vi "Dashboard Main.vi"() -> ()   [LabVIEW 2014]
uses:
  <vilib>/event_ctls.llb/eventvkey.ctl
  <vilib>/Rock Robotics/WPI/Dashboard/WPI_DashboardLogging Global.vi
  <vilib>/Utility/config.llb/Write Key (String).vi
  <vilib>/Utility/config.llb/Write Key (I32).vi
  <vilib>/Utility/config.llb/NI_LVConfig.lvlib
panel:
  out "Camera Image":T1(plugin-control)
  in  "TCP":refnum<k5>
  in  "Rec Mode":enum32{"Stop", "Record", "Playback"}(radio)
  in  "Vision":u16(ring) items=["Camera Off", "USB Camera SW", "USB Camera HW", "IP Camera"]
  out "Camera IP":string
  out "Image Message":string="Timeout in Camera Communications"
  in  "Dashboard Tab":T2(tab)
  in  "Drivetrain D":dbl
  in  "Drivetrain I":dbl
  in  "Drivetrain P":dbl
  in  "Camera Settings":T3={"Frame Rate"=30, "Compression"=30, "Size"=1} {"Frame Rate" scale=1.0..30.0; "Size" items=["640x480", "320x240", "160x120"]}
  out "MotorChart R":cluster{"Numeric":dbl, "Numeric":dbl}(graph)
  out "MotorChart L":T4(graph)
  out "MotorSliders R":cluster{"MotorSlide1":dbl, "MotorSlide2":dbl} {"MotorSlide2" scale=-1.0..1.0 scale format="%#_2e"; "MotorSlide1" scale=-1.0..1.0 scale format="%#_2e"}
  out "MotorSliders L":T5 {"MotorSlide4 2" scale=0.0..14.0 scale format="%#_2e"; "MotorSlide2" scale=-1.0..1.0 scale format="%#_2e"; "MotorSlide1" scale=-1.0..1.0 scale format="%#_2e"}
  out "Gyro":dbl(knob) scale=0.0..360.0
  out "JS1 Z":dbl(slide) scale=-1.0..1.0 scale format="%#_2e"
  out "JS1 Graph":cluster{"X":dbl, "Y":dbl}[](graph)
  out "JS1 Buttons":T6
  out "JS2 Z":dbl(slide) scale=-1.0..1.0 scale format="%#_2e"
  out "JS2 Graph":cluster{"X":dbl, "Y":dbl}[](graph)
  out "JS2 Buttons":T6
  out "Mode":T7(ring)=enum."Auto Disabled"
  in  "DB Camera Config":bool
  out "fps":dbl format="%#.1g"
  out "Mbps":dbl format="%#.1g"
  out "Mbps 2":bool
  in  "Test Slider":dbl(slide) scale=0.0..100.0 scale format="%#_3g"
  in  "On/Off":bool caption="Solenoid"
  in  "Test Name":u16(ring) items=["Select the test to run...", "Example Test", "-------------------------------", "List of tests is built in robot code.", "Replace with your own automated tests."]
  in  "Test Tree":string(tree)
  in  "Motor":cluster{"Value":dbl, "Enable":bool} {"Value" scale=-1.0..1.0 scale format="%#_3g"}
  out "Progress":T8 {"Test Progress" scale=0.0..100.0}
  in  "Rev/Fwd":cluster{"Forward":bool, "Reverse":bool}
  in  "Test Ring":u16(ring) items=["Monochrome", "Color"]
  in  "Listbox":i32(listbox)
  out "Tree":string(tree)
  # "Left"
  # "Front"
  # "Right"
  # "Battery"
  # "This tab is a great place for autonomous settings and robot-specific values.\nPlace controls and indicators inside this tab and match name to\nDashboard Variables on robot. You can also delete this comment."
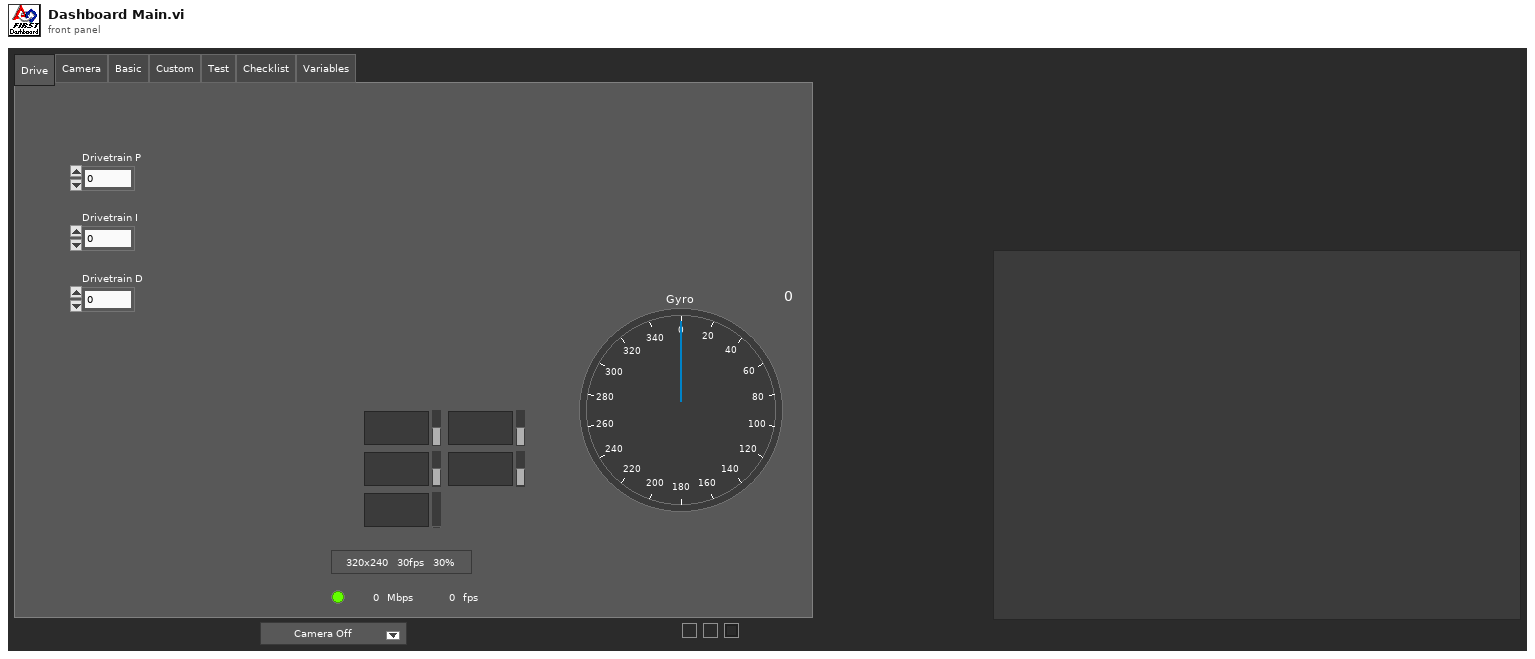
[diagram p1: front panel]
types:
  T1 = typedef "IMAQ Image.ctl" = refnum<image>
  T2 = enum32{"Drive", "Camera", "Basic", "Custom", "Test", "Checklist", "Variables"}
  T3 = cluster{"Frame Rate":i32, "Compression":i32, "Size":u16}
  T4 = cluster{"Numeric":dbl, "Numeric":dbl, "Battery V":dbl}
  T5 = cluster{"MotorSlide1":dbl, "MotorSlide2":dbl, "MotorSlide4 2":dbl}
  T6 = cluster{bool, bool, bool, bool, bool, bool, bool, bool, bool, bool, bool, bool}
  T7 = enum8{"Tele-Op Disabled", "Tele-Op Enabled", "Auto Disabled", "Auto Enabled", "Test Disabled", "Test Enabled", "Disconnected", "No Code", "E-Stop"}
  T8 = cluster{"Test Progress":u8, "Test Progress Text":string}
  T9 = typedef "Image Type" = u32
  T10 = cluster{"Error Strings":string, "Disable Counts":cluster{u16, u16}, "Rail Faults":cluster{u16, u16, u16}, "Robot IP":string, "DB Mode":u8, "Event Info":cluster{"Name":string, "Type":u8, "Number":u16, "Replay":u8}, "Camera Addr":string}
  T11 = cluster{"Storage":cluster{"Disk Free":u64, "RAM Block":u32, "RAM free":u32}, "CPU Utilization":cluster{"CPU % ISR":sgl, "CPU % Time Crit":sgl, "CPU % Timed Str":sgl, "CPU % High":sgl, "CPU % Above":sgl, "CPU % Normal":sgl, "CPU % Low":sgl}, "CAN":cluster{"% Bus Utilization":sgl, "Bus Off Cnt":u32, "TX_FIFO Full Cnt":u32, "Receive Error Cnt":u8, "Transmit Error Cnt":u8}, "HID":cluster{"HID Outputs":u32, "Rumble Low":u16, "Rumble High":u16}[]}
  T12 = cluster{"Status bits":cluster{"Test Mode":bool, "Autonomous":bool, "Enabled":bool, "Code Start":bool, "Brownout":bool, "Reserved 2":bool, "Reserved 3":bool, "E-Stop":bool}, "Code Trace":cluster{"Disabled":bool, "TeleOp":bool, "Auto":bool, "Test":bool}, "Controller Type":enum16{"unknown", "cRIO", "roboRio"}, "Code?":enum16{"unknown", "noCode", "code"}, "Battery V":dbl}
  T13 = cluster{"Control Bits":cluster{"TestMode":bool, "Autonomous":bool, "Enabled":bool, "FMS Present":bool, bool, bool, bool, "E-Stop":bool}, "Team Station ":u8, "Countdown":sgl, "Joystick Values":cluster{"Axes":dbl[], "Buttons":bool[], "POVs":i16[]}[]}
  T14 = cluster{"Axes":dbl[], "Buttons":bool[], "POVs":i16[]}[]
  T15 = cluster{"Axes":dbl[], "Buttons":bool[], "POVs":i16[]}
  T16 = cluster{"Buttons[0]":bool, "Buttons[1]":bool, "Buttons[2]":bool, "Buttons[3]":bool, "Buttons[4]":bool, "Buttons[5]":bool, "Buttons[6]":bool, "Buttons[7]":bool, "Buttons[8]":bool, "Buttons[9]":bool, "Buttons[10]":bool, "Buttons[11]":bool}
  T17 = typedef "NI_LVConfig.lvlib/Config Data RefNum.ctl" = refnum<k1>
  T18 = cluster{"Operation":enum16{"Update", "Clear"}, "Color Box":u32}[]
  T19 = typedef "eventvkey.ctl" = enum16{"ASCII", "Enter", "Return", "Shift", "Ctrl", "Alt", "Cmd", "Opt", "Caps", "NumLock", "Clear", "Break", "Up", "Down", "Left", "Right", "Insert", "Delete", "Home", "End", "PageUp", "PageDown", "Escape", "Help", "Pause", "ScrollLock", "F1", "F2", "F3", "F4", "F5", "F6", "F7", "F8", "F9", "F10", "F11", "F12", "F13", "F14", "F15", "F16", "F17", "F18", "F19", "F20", "F21", "F22", "F23", "F24", "Play", "VolumeUp", "VolumeDown", "Mute", "Two Byte Char"}
  T20 = cluster{"Image Size":bool, "Image Type":bool, "Pixel Value":bool, "ROI Information":bool, "Zoom Factor":bool}
  T21 = enum8{"Enabled", "Disabled", "Disabled and Grayed Out"}
  T22 = cluster{"Operation":enum16{"Update", "Clear"}, "Color Box":u32}
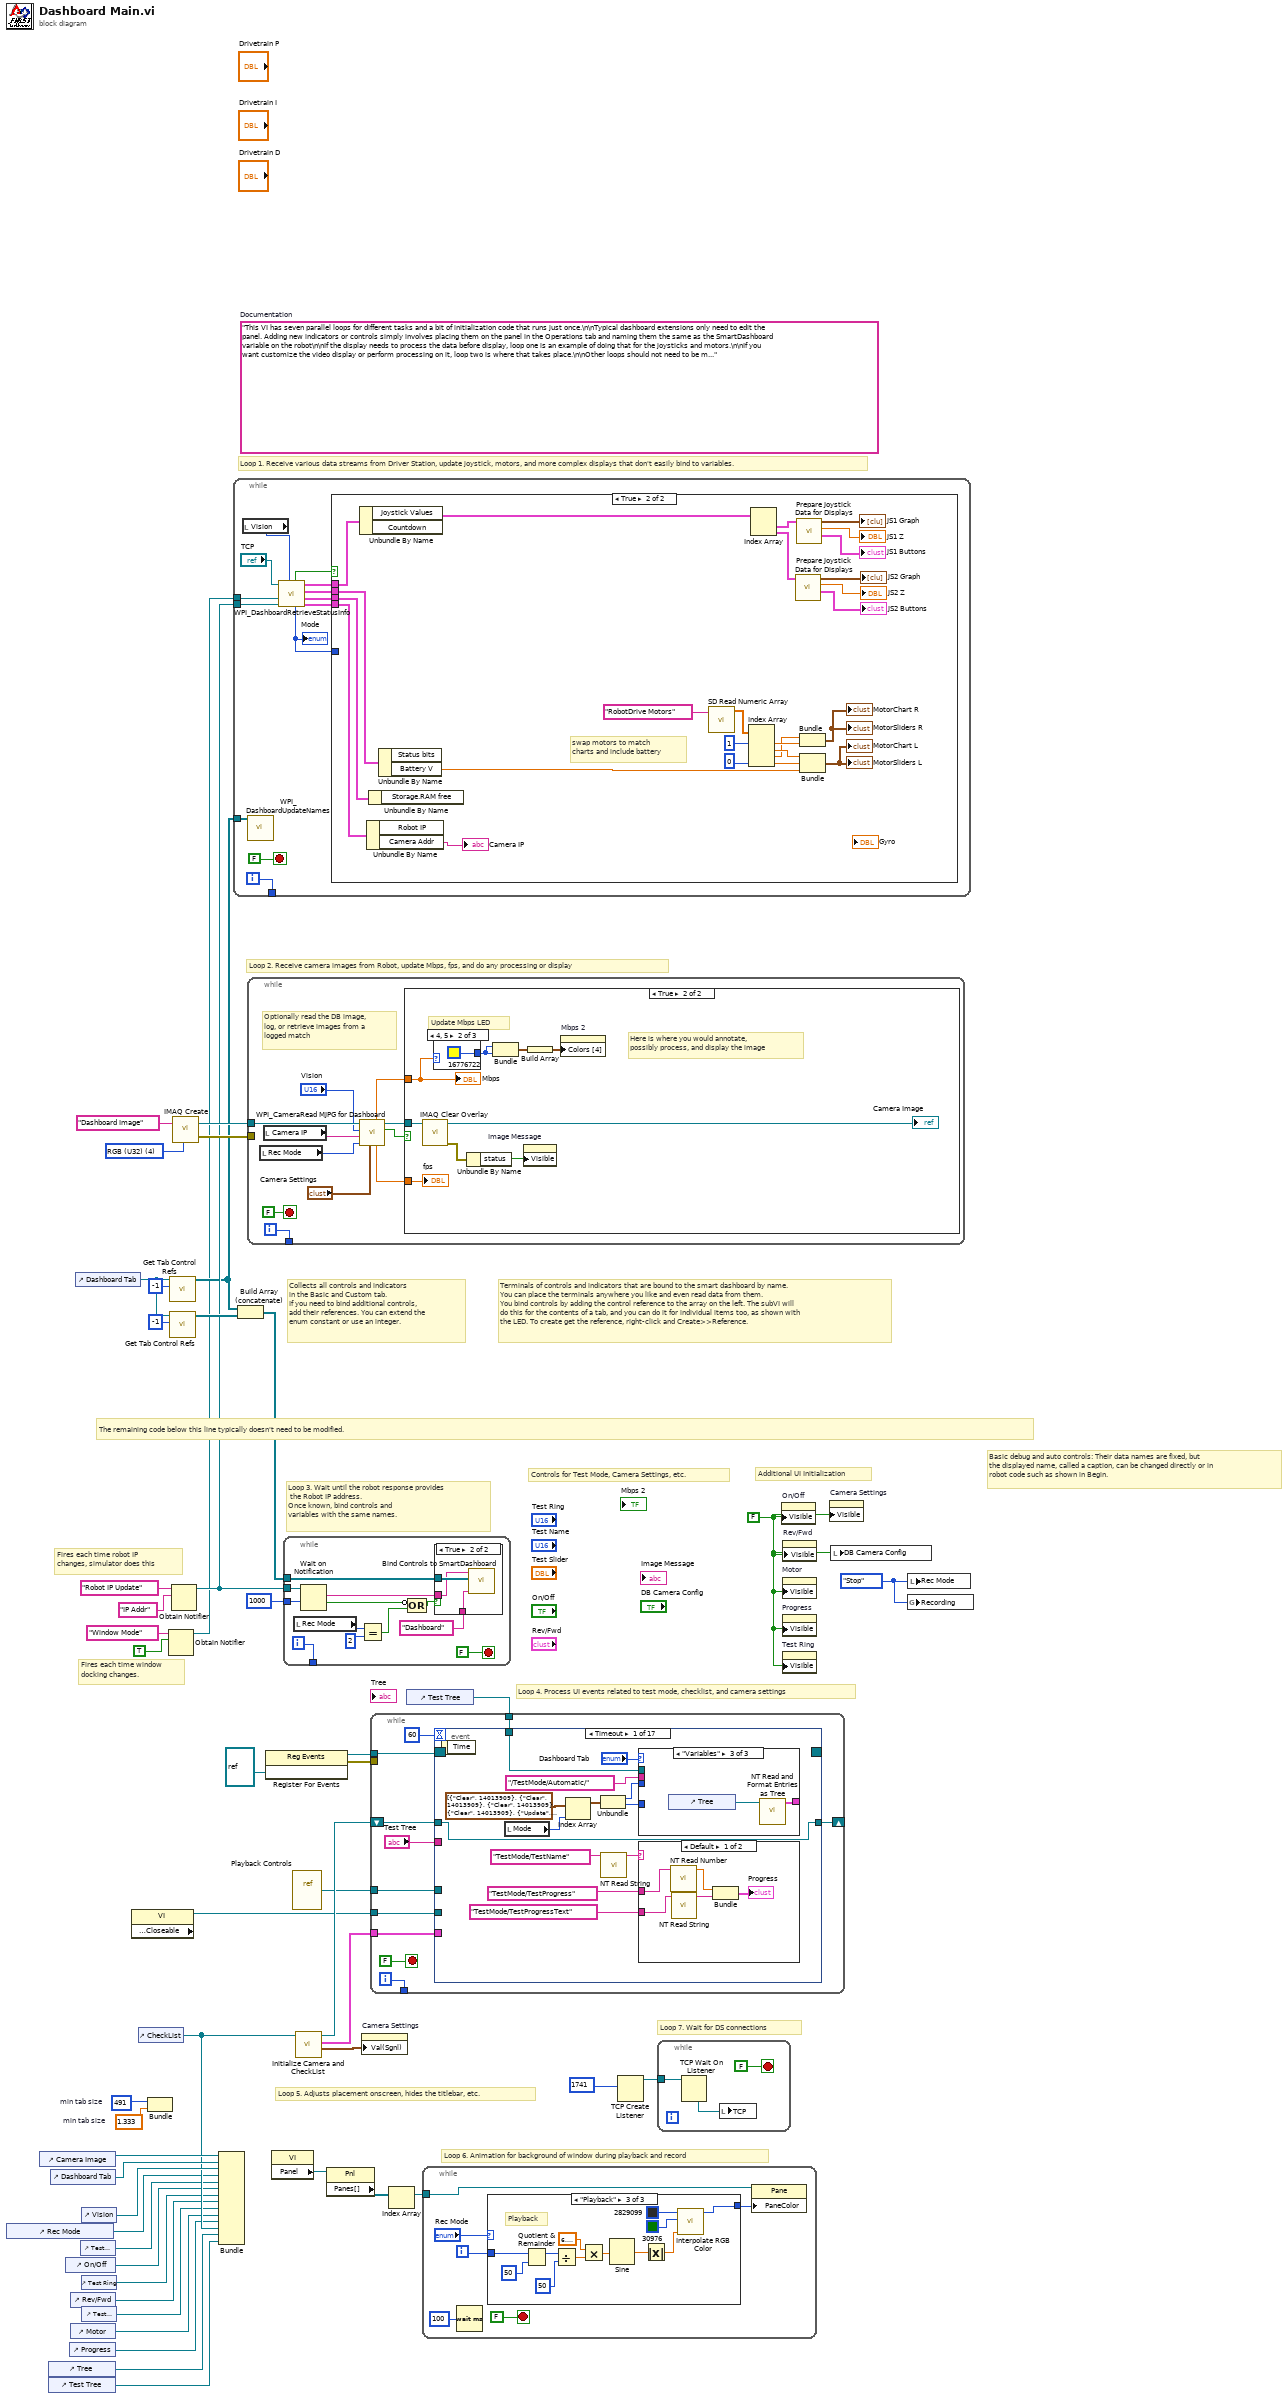
[diagram p0: block diagram]
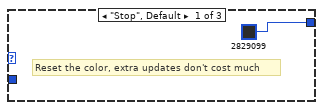
[diagram p3: hidden frame]
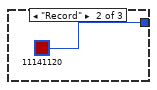
[diagram p4: hidden frame]
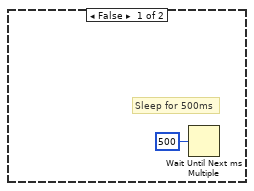
[diagram p6: hidden frame]
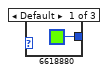
[diagram p7: hidden frame]
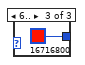
[diagram p8: hidden frame]
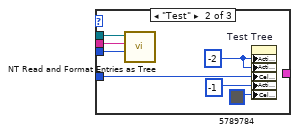
[diagram p10: hidden frame]
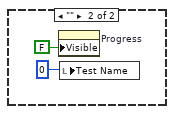
[diagram p11: hidden frame]
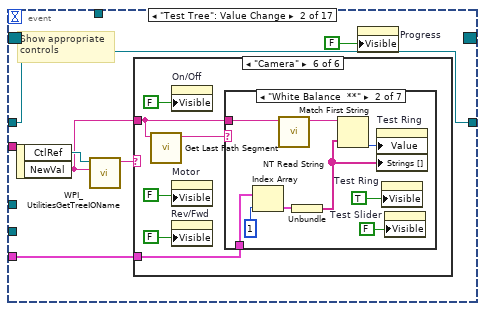
[diagram p12: hidden frame]
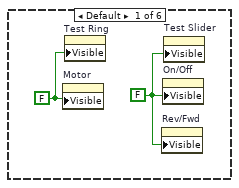
[diagram p13: hidden frame]
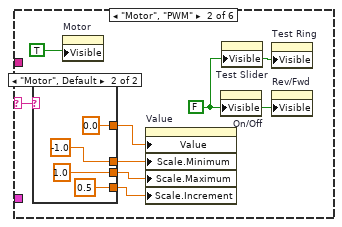
[diagram p14: hidden frame]
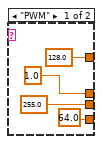
[diagram p15: hidden frame]
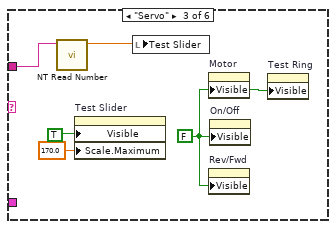
[diagram p16: hidden frame]
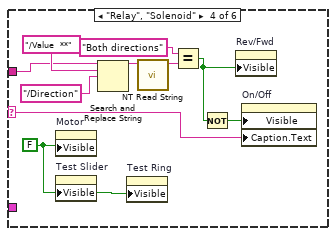
[diagram p17: hidden frame]
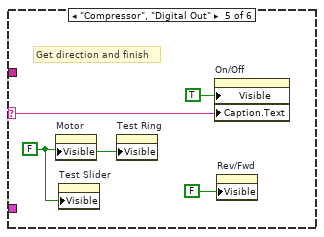
[diagram p18: hidden frame]
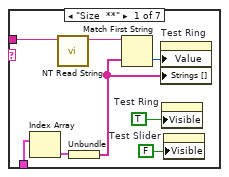
[diagram p19: hidden frame]
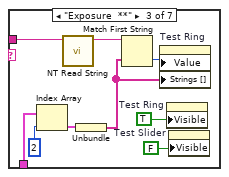
[diagram p20: hidden frame]
diagram:
  w21 = 491  # min tab size
  w20 = 1.333  # min tab size
  w29 = enum32{"Stop", "Record", "Playback"}."Stop" ("Rec Mode")
  w8 = FALSE ("Visible")
  (unwired) "This VI has seven parallel loops for different tasks and a bit of initialization code that runs just once.\n\nTypical dashboard extensions only need to edit the panel. Adding new indicators or controls simply involves placing them on the panel in the Operations tab and naming them the same as the SmartDashboard variable on the robot\n\nIf the display needs to process the data before display, loop one is an example of doing that for the joysticks and motors.\n\nIf you want customize the video display or perform processing on it, loop two is where that takes place.\n\nOther loops should not need to be modified. They are pretty standard, and document the task they perform."  # Documentation
  w49 = T9 4 items=["Grayscale (U8)", "Grayscale (I16)", "Grayscale (SGL)", "Complex (CSG)", "RGB (U32)", "HSL (U32)", "RGB (U64)"] ("Image Type")
  # "Loop 7. Wait for DS connections"
  # "Basic debug and auto controls: Their data names are fixed, but\nthe displayed name, called a caption, can be changed directly or in\nrobot code such as shown in Begin."
  # "Controls for Test Mode, Camera Settings, etc."
  # "Additional UI Initialization"
  # "Loop 6. Animation for background of window during playback and record"
  # "Fires each time robot IP\nchanges, simulator does this"
  # "Fires each time window\ndocking changes."
  # "Collects all controls and indicators\nin the Basic and Custom tab.\nIf you need to bind additional controls,\nadd their references. You can extend the\nenum constant or use an integer."
  # "The remaining code below this line typically doesn't need to be modified."
  # "Loop 4. Process UI events related to test mode, checklist, and camera settings"
  # "Terminals of controls and indicators that are bound to the smart dashboard by name.\nYou can place the terminals anywhere you like and even read data from them.\nYou bind controls by adding the control reference to the array on the left. The subVI will\ndo this for the contents of a tab, and you can do it for individual items too, as shown with\nthe LED. To create get the reference, right-click and Create>>Reference."
  # "Loop 3. Wait until the robot response provides\n the Robot IP address.\nOnce known, bind controls and\nvariables with the same names."
  # "Loop 5. Adjusts placement onscreen, hides the titlebar, etc."
  # "Loop 1. Receive various data streams from Driver Station, update joystick, motors, and more complex displays that don't easily bind to variables."
  # "Loop 2. Receive camera images from Robot, update Mbps, fps, and do any processing or display"
  n1 = control-ref of="Rec Mode"() -> (w14:refnum<vi>)
  n2 = control-ref of="Camera Image"() -> (w24:refnum<vi>)
  n3 = control-ref of="Tree"() -> (w18:refnum<vi>)
  n4 = control-ref of="Test Tree"() -> (w17:refnum<vi>)
  n5 = control-ref of="Dashboard Tab"() -> (w23:refnum<vi>)
  n6 = control-ref of="On/Off"() -> (w12:refnum<vi>)
  n7 = control-ref of="Progress"() -> (w9:refnum<vi>)
  n8 = control-ref of="Rev/Fwd"() -> (w10:refnum<vi>)
  n9 = control-ref of="Motor"() -> (w15:refnum<vi>)
  n10 = control-ref of="Dashboard Tab"() -> (w27:refnum<vi>)
  n11 = control-ref of="Test Slider"() -> (w13:refnum<vi>)
  n12 = control-ref of="Vision"() -> (w22:refnum<vi>)
  n13 = control-ref of="Test Ring"() -> (w11:refnum<vi>)
  n14 = control-ref of="Test Name"() -> (w16:refnum<vi>)
  n15 = property class="VI" props=["Front Panel.Closeable"]() -> (reference out=w28:refnum<vi>)  [unwired: 2 in, 2 out]
  n16 = control-ref of="CheckList"() -> (w19:refnum<vi>)
  n17 = Bundle("min tab size"=w21, "min tab size"=w20) -> ()  [unwired: 1 in, 1 out]
  n18 = Obtain Notifier(name (unnamed)="Window Mode", notification data type=TRUE) -> (notifier out=w5:refnum<notifier>)  [unwired: 2 in, 2 out]
  n19 = call <vilib>:"Get Tab Control Refs.vi"("Page Index"=-1, "TabControl in"=w27) -> ("ControlsOnPage"=w6:refnum<vi>[])  [unwired: 9 in]
  n20 = call <vilib>:"Get Tab Control Refs.vi"("Page Index"=-1, "TabControl in"=w27) -> ("ControlsOnPage"=w26:refnum<vi>[])  [unwired: 9 in]
  n21 = Obtain Notifier(name (unnamed)="Robot IP Update", notification data type="IP Addr" ("name (unnamed)")) -> (notifier out=w7:refnum<notifier>)  [unwired: 2 in, 2 out]
  n22 = call "IMAQ Create"("Image Name"="Dashboard Image", "Image Type"=w49) -> ("New Image"=w47:T1, "error out"=w46:errorcluster)  [unwired: 2 in, 1 out]
  n23 = Bundle("Camera Image"=w24, "Dashboard Tab"=w23, "Vision"=w22, "Rec Mode"=w14, "Test Slider"=w13, "On/Off"=w12, "Test Ring"=w11, "Rev/Fwd"=w10, "Test Name"=w16, "Motor"=w15, "Progress"=w9, "CheckList"=w19, "Tree"=w18, "Test Tree"=w17) -> ()  [unwired: 1 in, 1 out]
  n24 = while {
    tunnel: [w61] -> _
    tunnel: w7 -> [w55]
    tunnel: w6 -> [w54]
    tunnel: w5 -> [w50]
    i -> [w61]
    stop <- FALSE stop-if-true
    n25 = local read "Vision"() -> (w52:u16)
    n26 = call <vilib>:"WPI_DashboardUpdateNames.vi"("Controls on Tab"=w54) -> ()  [unwired: 11 in]
    n27 = call <vilib>:"WPI_DashboardRetrieveStatusInfo.vi"("Vision"=w52, "Binding Refnum"=w55, "Window Mode Notifier"=w50, "TCP Cnx"="TCP") -> ("Power and Errors"=w56:T10, "Robot Metrics"=w59:T11, "Status Info"=w60:T12, "Control Info"=w57:T13, "Robot Mode"=w53:T7, "Process?"=w58:bool)  [unwired: 2 in]
    "Mode" <- w53
    n28 = case shown="True" w58 {
      tunnel: w60 -> [_ w87]
      tunnel: w59 -> [_ w86]
      tunnel: w57 -> [_ w85]
      tunnel: w56 -> [_ w84]
      tunnel: w53 -> [_ _]
      frame False {
      }
      frame True {
        # "swap motors to match\ncharts and include battery"
        n29 = Unbundle By Name(w85) -> ("Joystick Values"=w72:T14)  [unwired: 1 out]
        n30 = Unbundle By Name(w84) -> ("Camera Addr"=→"Camera IP":string)  [unwired: 1 out]
        n31 = Unbundle By Name(w86) -> ()  [unwired: 1 out]
        n32 = Unbundle By Name(w87) -> ("Battery V"=w73:dbl)  [unwired: 1 out]
        n33 = call <vilib>:"SD Read Numeric Array.vi"("Name"="RobotDrive Motors") -> ("Numeric Array"=w75:dbl[])  [unwired: 8 in, 2 out]
        n34 = Index Array(array=w75, index #1=1, index #4=0) -> (element #1=w79:dbl, element #2=w80:dbl, element #3=w78:dbl, element #4=w83:dbl)  [unwired: 2 in]
        n35 = Index Array(array=w72) -> (element #1=w71:T15, element #2=w66:T15)  [unwired: 2 in]
        n36 = call "Prepare Joystick Data for Displays.vi"("Joystick Values"=w66) -> ("Buttons"=→"JS2 Buttons":T16, "Z Axis"=→"JS2 Z":dbl, "Cartesian Data"=→"JS2 Graph":cluster{"X axis":dbl, "X axis":dbl}[])  [unwired: 8 in]
        n37 = call "Prepare Joystick Data for Displays.vi"("Joystick Values"=w71) -> ("Buttons"=→"JS1 Buttons":T16, "Z Axis"=→"JS1 Z":dbl, "Cartesian Data"=→"JS1 Graph":cluster{"X axis":dbl, "X axis":dbl}[])  [unwired: 8 in]
        n38 = Bundle("Numeric"=w78, "Numeric"=w79) -> (→"MotorChart R" →"MotorSliders R":cluster{"Numeric":dbl, "Numeric":dbl})  [unwired: 1 in]
        n39 = Bundle("Numeric"=w80, "Numeric"=w83, "Battery V"=w73) -> (→"MotorChart L" →"MotorSliders L":T4)  [unwired: 1 in]
      }
    }
  }
  n40 = Build Array (concatenate)(w6, w26) -> (w25:refnum<vi>[])
  n41 = while {
    tunnel: w47 -> [w96]
    tunnel: w46 -> [_]
    tunnel: [w97] -> _
    i -> [w97]
    stop <- FALSE stop-if-true
    # "Optionally read the DB image,\nlog, or retrieve images from a\nlogged match"
    n42 = local read "Rec Mode"() -> (w90:enum32{"Stop", "Record", "Playback"})
    n43 = local read "Camera IP"() -> (w88:string)
    n44 = call <vilib>:"WPI_CameraRead MJPG for Dashboard.vi"("Camera Settings"="Camera Settings", "Rec Mode"=w90, "Camera IP"=w88, "Camera Mode"="Vision", "Refnum in"=w96) -> ("Active"=w94:bool, "Refnum out"=w95:T1, "FPS"=w93:dbl, "Bandwidth (Mbps)"=w92:dbl)  [unwired: 3 in]
    n45 = case shown="True" w94 {
      tunnel: w95 -> [_ w103]
      tunnel: w92 -> [_ w102]
      tunnel: w93 -> [_ w100]
      frame False {
        # "Sleep for 500ms"
        n46 = Wait Until Next ms Multiple(millisecond multiple=u32 500) -> ()  [unwired: 1 out]
      }
      frame True {
        # "Here is where you would annotate,\npossibly process, and display the image"
        # "Update Mbps LED"
        n47 = call "IMAQ Clear Overlay"("Image"=w103) -> ("error out"=w107:errorcluster, "Image Out"=→"Camera Image":T1)  [unwired: 2 in, 7 out]
        n48 = case shown="4, 5" w102 {
          tunnel: [u32 6618880 ("Color Box") u32 16776722 ("Color Box") u32 16716800 ("Color Box")] -> w104
          frame Default {
          }
          frame 4, 5 {
          }
          frame 6.. {
          }
        }
        n49 = Unbundle By Name(w107) -> ("status"=w108:bool)
        n50 = Bundle("Color Box"=w104, "Color Box"=w104) -> (w106:cluster{"Color Box":u32, "Color Box":u32})  [unwired: 1 out]
        n51 = property on="Image Message" class="Str"("Visible"=w108) -> ()  [unwired: 2 in, 2 out]
        n52 = Build Array(w106) -> (w105:cluster{"Color Box":u32, "Color Box":u32}[])
        n53 = property on="Mbps 2" class="Bool (strict)"("Colors [4]"=w105) -> ()  [unwired: 2 in, 2 out]
        "Mbps" <- w102
        "fps" <- w100
      }
    }
  }
  n54 = register-events(refnum<vi> refnum) -> (reference out=w33:refnum<event-registration>, error out=w32:errorcluster)  [unwired: 2 in]
  n55 = property class="VI"() -> ("Panel"=w36:refnum<vi>)  [unwired: 2 in, 2 out]
  n56 = while {
    tunnel: w25 -> [w123]
    tunnel: w7 -> [w121]
    tunnel: [w119] -> _
    tunnel: u32 1000 ("milliseconds to wait") -> [w118]
    i -> [w119]
    stop <- FALSE stop-if-true
    n57 = local read "Rec Mode"() -> (w114:enum32{"Stop", "Record", "Playback"})
    n58 = Wait on Notification(notifier=w121, timeout in ms (-1)=w118) -> (notification=w120:string, timed out?=w116:bool)  [unwired: 2 in, 2 out]
    n59 = Equal?(x=w114, y=u16 2 ("Rec Mode")) -> (x = y?=w115:bool)
    n60 = Compound Arithmetic op=OR(invert w116, w115) -> (w117:bool)
    n61 = case shown="True" w117 {
      tunnel: w123 -> [_ w126]
      tunnel: w120 -> [_ w125]
      tunnel: "Dashboard" -> [_ w124]
      frame False {
      }
      frame True {
        n62 = call <vilib>:"Bind Controls to SmartDashboard.vi"("Client Name"=w124, "Bound Control Refs"=w126, "Server IP Address"=w125) -> ()  [unwired: 9 in]
      }
    }
  }
  n63 = vi-ref "Playback Controls.vi"() -> (w34:refnum<vi>)
  n64 = call "Initialize Camera and CheckList.vi"("ListBox in"=w19) -> ("Cluster"=w40:cluster{"value":i32, "value":i32, "index":i32}, "Array"=w41:cluster{string[]}[], "File Refnum"=w39:T17)  [unwired: 8 in]
  n65 = property class="Pnl"(reference=w36) -> ("Panes[]"=w37:refnum<vi>[])  [unwired: 1 in, 2 out]
  n66 = property on="Camera Settings" class="Clust (strict)"("Val(Sgnl)"=w40) -> ()  [unwired: 2 in, 2 out]
  n67 = Index Array(array=w37) -> (element=w35:refnum<vi>)  [unwired: 1 in]
  n68 = control-ref of="Test Tree"() -> (w38:refnum<vi>)
  n69 = while {
    tunnel: w41 -> [w134]
    shift-right: [w133] -> _
    shift-left: w39 -> [w132]
    tunnel: [w131] -> _
    tunnel: w38 -> [w130]
    tunnel: w34 -> [w129]
    tunnel: w33 -> [w128]
    tunnel: w32 -> [_]
    tunnel: w28 -> [w127]
    i -> [w131]
    stop <- FALSE stop-if-true
    n70 = event shown="[0] Timeout" {
      selector: w128 -> [_ _ _ _ _ _ _ _ _ _ _ _ _ _ _ _ _]
      dyn-events: [_ _ _ _ _ _ _ _ _ _ _ _ _ w372 _ _ _] -> _
      timeout: u32 60 ("milliseconds to wait") -> [_ _ _ _ _ _ _ _ _ _ _ _ _ _ _ _ _]
      tunnel: w130 -> [w146 _ _ _ _ _ _ _ _ _ _ _ _ _ _ _ _]
      tunnel: "Test Tree" -> [_ _ _ _ _ _ _ _ w341 w349 w351 w355 w363 _ _ _ _]
      tunnel: w134 -> [_ w168 _ _ _ _ w305 w335 _ _ _ _ _ _ _ _ _]
      tunnel: [w142 w167 w266 w271 w279 w291 w304 w328 w340 w347 w350 w354 w362 w374 w388 w389 w399] -> w133
      tunnel: w132 -> [w142 w167 w266 w271 w279 w291 w303 w328 w340 w347 w350 w354 w362 w374 w388 w389 w399]
      tunnel: w129 -> [_ _ _ _ _ _ _ _ _ _ _ _ _ w375 _ w392 _]
      tunnel: w127 -> [_ _ _ _ _ _ _ _ _ _ _ _ _ w370 _ _ _]
      event Timeout {
        n71 = event-data() -> ()  [unwired: 1 in, 1 out]
        n72 = local read "Mode"() -> (w145:T7)
        n73 = Index Array(array=T18 [{"Operation"=enum."Clear", "Color Box"=14013909}, {"Operation"=enum."Clear", "Color Box"=14013909}, {"Operation"=enum."Clear", "Color Box"=14013909}, {"Operation"=enum."Clear", "Color Box"=14013909}, {"Operation"=enum."Update", "Color Box"=14013909}, {"Operation"=enum."Update", "Color Box"=16777215}, {"Operation"=enum."Clear", "Color Box"=14013909}, {"Operation"=enum."Clear", "Color Box"=14013909}, {"Operation"=enum."Clear", "Color Box"=14013909}], index=w145) -> (element=w140:T22)
        n74 = Unbundle(w140) -> ("Operation"=w139:enum16{"Update", "Clear"}, "Color Box"=w138:u32)
        n75 = call <vilib>:"NT Read String.vi"("Name"="TestMode/TestName") -> ("String"=w149:string)  [unwired: 9 in, 1 out]
        n76 = case shown="\"Variables\"" "Dashboard Tab" {
          tunnel: w146 -> [_ w157 _]
          tunnel: "/TestMode/Automatic/" ("Name Pattern") -> [_ w156 _]
          tunnel: w139 -> [_ w155 _]
          tunnel: [_ _ w159] -> _
          tunnel: w138 -> [_ w151 _]
          frame "Custom", Default {
          }
          frame "Test" {
            w154 = -2 ("Active Item:Row Number")
            n77 = call <vilib>:"NT Read and Format Entries as Tree.vi"("Operation"=w155, "Name Pattern"=w156, "Tree Refnum"=w157) -> ()  [unwired: 7 in, 2 out]
            n78 = property on="Test Tree" class="Tree (strict)"("Active Item Row Number"=w154, "ActiveColNum"=w154, "CellBG"=w151, "Active Item Row Number"=-1 ("Active Item:Row Number"), "CellBG"=u32 5789784 ("Color Box")) -> ()  [unwired: 2 in, 2 out]
          }
          frame "Variables" {
            n79 = control-ref of="Tree"() -> (w158:refnum<vi>)
            n80 = call <vilib>:"NT Read and Format Entries as Tree.vi"("Tree Refnum"=w158) -> ("Formatted Strings"=w159:cluster{"Name":string, "Value":string}[])  [unwired: 9 in, 1 out]
          }
        }
        n81 = case shown="Default" w149 {
          tunnel: "TestMode/TestProgress" ("Name") -> [w161 _]
          tunnel: "TestMode/TestProgressText" ("Name") -> [w160 _]
          frame Default {
            n82 = call <vilib>:"NT Read Number.vi"("Name"=w161) -> ("Numeric"=w162:dbl)  [unwired: 9 in, 1 out]
            n83 = call <vilib>:"NT Read String.vi"("Name"=w160) -> ("String"=w163:string)  [unwired: 9 in, 1 out]
            n84 = Bundle("Numeric"=w162, "String"=w163) -> (→"Progress":cluster{"Numeric":dbl, "String":string})  [unwired: 1 in]
          }
          frame "" {
            n85 = property on="Progress" class="Clust (strict)"("Visible"=FALSE) -> ()  [unwired: 2 in, 2 out]
            n86 = local write "Test Name"(u16 0) -> ()
          }
        }
      }
      event "Test Tree": Value Change {
        # "Show appropriate\ncontrols"
        n87 = event-data() -> ("CtlRef"=w171:refnum<vi>, "NewVal"=w169:string)  [unwired: 1 in]
        n88 = call <vilib>:"WPI_UtilitiesGetTreeIOName.vi"("NewVal"=w169, "TreeControl in"=w171) -> ("I/O Name"=w172:string)  [unwired: 9 in]
        n89 = case shown="\"Camera\"" w172 {
          selector: w172 -> [_ w179 _ w197 w206 _]
          tunnel: w169 -> [_ _ w194 w196 _ w213]
          tunnel: w168 -> [_ _ _ _ _ w212]
          frame Default {
            w174 = FALSE ("Visible")
            w173 = FALSE ("Visible")
            n90 = property on="Motor" class="Clust (strict)"("Visible"=w173) -> ()  [unwired: 2 in, 2 out]
            n91 = property on="Test Ring" class="Ring (strict)"("Visible"=w173) -> ()  [unwired: 2 in, 2 out]
            n92 = property on="Rev/Fwd" class="Clust (strict)"("Visible"=w174) -> ()  [unwired: 2 in, 2 out]
            n93 = property on="On/Off" class="Bool (strict)"("Visible"=w174) -> ()  [unwired: 2 in, 2 out]
            n94 = property on="Test Slider" class="Slide (strict)"("Visible"=w174) -> ()  [unwired: 2 in, 2 out]
          }
          frame "Motor", "PWM" {
            w180 = FALSE ("Visible")
            n95 = case shown="\"Motor\", Default" w179 {
              tunnel: [1.0 ("Value") -1.0 ("Value")] -> w178
              tunnel: [255.0 ("Value") 1.0 ("Value")] -> w177
              tunnel: [128.0 ("Value") 0.0 ("Value")] -> w176
              tunnel: [64.0 ("Value") 0.5 ("Value")] -> w175
              frame "PWM" {
              }
              frame "Motor", Default {
              }
            }
            n96 = property on="Motor" class="Clust (strict)"("Visible"=TRUE) -> ()  [unwired: 2 in, 2 out]
            n97 = property on="Value" class="Slide (strict)"("Value"=w176, "Scale.Minimum"=w178, "Scale.Maximum"=w177, "Scale.Increment"=w175) -> ()  [unwired: 2 in, 2 out]
            n98 = property on="On/Off" class="Bool (strict)"("Visible"=w180) -> ()  [unwired: 2 in, 2 out]
            n99 = property on="Test Slider" class="Slide (strict)"("Visible"=w180) -> ()  [unwired: 2 in, 2 out]
            n100 = property on="Test Ring" class="Ring (strict)"("Visible"=w180) -> ()  [unwired: 2 in, 2 out]
            n101 = property on="Rev/Fwd" class="Clust (strict)"("Visible"=w180) -> ()  [unwired: 2 in, 2 out]
          }
          frame "Servo" {
            w192 = FALSE ("Visible")
            n102 = call <vilib>:"NT Read Number.vi"("Name"=w194) -> ("Numeric"=w193:dbl)  [unwired: 9 in, 1 out]
            n103 = property on="Test Slider" class="Slide (strict)"("Visible"=TRUE, "Scale.Maximum"=170.0 ("Scale.Range:Maximum")) -> ()  [unwired: 2 in, 2 out]
            n104 = local write "Test Slider"(w193) -> ()
            n105 = property on="Motor" class="Clust (strict)"("Visible"=w192) -> ()  [unwired: 2 in, 2 out]
            n106 = property on="Rev/Fwd" class="Clust (strict)"("Visible"=w192) -> ()  [unwired: 2 in, 2 out]
            n107 = property on="On/Off" class="Bool (strict)"("Visible"=w192) -> ()  [unwired: 2 in, 2 out]
            n108 = property on="Test Ring" class="Ring (strict)"("Visible"=w192) -> ()  [unwired: 2 in, 2 out]
          }
          frame "Relay", "Solenoid" {
            w195 = FALSE ("Visible")
            n109 = property on="Motor" class="Clust (strict)"("Visible"=w195) -> ()  [unwired: 2 in, 2 out]
            n110 = property on="Test Slider" class="Slide (strict)"("Visible"=w195) -> ()  [unwired: 2 in, 2 out]
            n111 = Search and Replace String(input string=w196, search string="/Value  **", replace string="/Direction") -> (result string=w202:string)  [unwired: 5 in, 3 out]
            n112 = property on="Test Ring" class="Ring (strict)"("Visible"=w195) -> ()  [unwired: 2 in, 2 out]
            n113 = call <vilib>:"NT Read String.vi"("Name"=w202) -> ("String"=w200:string)  [unwired: 9 in, 1 out]
            n114 = Equal?(x="Both directions", y=w200) -> (x = y?=w198:bool)
            n115 = Not(x=w198) -> (.not. x?=w199:bool)
            n116 = property on="Rev/Fwd" class="Clust (strict)"("Visible"=w198) -> ()  [unwired: 2 in, 2 out]
            n117 = property on="On/Off" class="Bool (strict)"("Visible"=w199, "Caption.Text"=w197) -> ()  [unwired: 2 in, 2 out]
          }
          frame "Compressor", "Digital Out" {
            w205 = FALSE ("Visible")
            # "Get direction and finish"
            n118 = property on="Motor" class="Clust (strict)"("Visible"=w205) -> ()  [unwired: 2 in, 2 out]
            n119 = property on="Test Slider" class="Slide (strict)"("Visible"=w205) -> ()  [unwired: 2 in, 2 out]
            n120 = property on="Test Ring" class="Ring (strict)"("Visible"=w205) -> ()  [unwired: 2 in, 2 out]
            n121 = property on="On/Off" class="Bool (strict)"("Visible"=TRUE, "Caption.Text"=w206) -> ()  [unwired: 2 in, 2 out]
            n122 = property on="Rev/Fwd" class="Clust (strict)"("Visible"=FALSE) -> ()  [unwired: 2 in, 2 out]
          }
          frame "Camera" {
            n123 = call <vilib>:"Get Last Path Segment.vi"("String in"=w213) -> ("String out"=w214:string)  [unwired: 10 in]
            n124 = property on="On/Off" class="Bool (strict)"("Visible"=FALSE) -> ()  [unwired: 2 in, 2 out]
            n125 = property on="Motor" class="Clust (strict)"("Visible"=FALSE) -> ()  [unwired: 2 in, 2 out]
            n126 = property on="Rev/Fwd" class="Clust (strict)"("Visible"=FALSE) -> ()  [unwired: 2 in, 2 out]
            n127 = case shown="\"White Balance  **\"" w214 {
              tunnel: w213 -> [w220 w229 w238 w247 w256 _ w262]
              tunnel: w212 -> [w218 w226 w235 w244 w253 _ _]
              frame "Size  **" {
                n128 = Index Array(array=w218) -> (element=w217:cluster{string[]})  [unwired: 1 in]
                n129 = call <vilib>:"NT Read String.vi"("Name"=w220) -> ("String"=w219:string)  [unwired: 9 in, 1 out]
                n130 = Unbundle(w217) -> (w215:string[])
                n131 = Match First String(2:w215, 3:w219) -> (0:w216:i32)  [unwired: 1 out]
                n132 = property on="Test Ring" class="Ring (strict)"("Value"=w216, "Strings []"=w215) -> ()  [unwired: 2 in, 2 out]
                n133 = property on="Test Ring" class="Ring (strict)"("Visible"=TRUE) -> ()  [unwired: 2 in, 2 out]
                n134 = property on="Test Slider" class="Slide (strict)"("Visible"=FALSE) -> ()  [unwired: 2 in, 2 out]
              }
              frame "White Balance  **" {
                n135 = Index Array(array=w226, index=1) -> (element=w227:cluster{string[]})
                n136 = call <vilib>:"NT Read String.vi"("Name"=w229) -> ("String"=w228:string)  [unwired: 9 in, 1 out]
                n137 = Unbundle(w227) -> (w224:string[])
                n138 = Match First String(2:w224, 3:w228) -> (0:w223:i32)  [unwired: 1 out]
                n139 = property on="Test Ring" class="Ring (strict)"("Value"=w223, "Strings []"=w224) -> ()  [unwired: 2 in, 2 out]
                n140 = property on="Test Ring" class="Ring (strict)"("Visible"=TRUE) -> ()  [unwired: 2 in, 2 out]
                n141 = property on="Test Slider" class="Slide (strict)"("Visible"=FALSE) -> ()  [unwired: 2 in, 2 out]
              }
              frame "Exposure  **" {
                n142 = Index Array(array=w235, index=2) -> (element=w236:cluster{string[]})
                n143 = call <vilib>:"NT Read String.vi"("Name"=w238) -> ("String"=w237:string)  [unwired: 9 in, 1 out]
                n144 = Unbundle(w236) -> (w232:string[])
                n145 = Match First String(2:w232, 3:w237) -> (0:w233:i32)  [unwired: 1 out]
                n146 = property on="Test Ring" class="Ring (strict)"("Value"=w233, "Strings []"=w232) -> ()  [unwired: 2 in, 2 out]
                n147 = property on="Test Ring" class="Ring (strict)"("Visible"=TRUE) -> ()  [unwired: 2 in, 2 out]
                n148 = property on="Test Slider" class="Slide (strict)"("Visible"=FALSE) -> ()  [unwired: 2 in, 2 out]
              }
              frame "Exposure Priority  **" {
                n149 = Index Array(array=w244, index=3) -> (element=w245:cluster{string[]})
                n150 = call <vilib>:"NT Read String.vi"("Name"=w247) -> ("String"=w246:string)  [unwired: 9 in, 1 out]
                n151 = Unbundle(w245) -> (w241:string[])
                n152 = Match First String(2:w241, 3:w246) -> (0:w242:i32)  [unwired: 1 out]
                n153 = property on="Test Ring" class="Ring (strict)"("Value"=w242, "Strings []"=w241) -> ()  [unwired: 2 in, 2 out]
                n154 = property on="Test Ring" class="Ring (strict)"("Visible"=TRUE) -> ()  [unwired: 2 in, 2 out]
                n155 = property on="Test Slider" class="Slide (strict)"("Visible"=FALSE) -> ()  [unwired: 2 in, 2 out]
              }
              frame "Color Enable  **" {
                n156 = Index Array(array=w253, index=4) -> (element=w254:cluster{string[]})
                n157 = call <vilib>:"NT Read String.vi"("Name"=w256) -> ("String"=w255:string)  [unwired: 9 in, 1 out]
                n158 = Unbundle(w254) -> (w250:string[])
                n159 = Match First String(2:w250, 3:w255) -> (0:w251:i32)  [unwired: 1 out]
                n160 = property on="Test Ring" class="Ring (strict)"("Value"=w251, "Strings []"=w250) -> ()  [unwired: 2 in, 2 out]
                n161 = property on="Test Ring" class="Ring (strict)"("Visible"=TRUE) -> ()  [unwired: 2 in, 2 out]
                n162 = property on="Test Slider" class="Slide (strict)"("Visible"=FALSE) -> ()  [unwired: 2 in, 2 out]
              }
              frame Default {
                n163 = property on="Test Ring" class="Ring (strict)"("Visible"=FALSE) -> ()  [unwired: 2 in, 2 out]
                n164 = property on="Test Slider" class="Slide (strict)"("Visible"=FALSE) -> ()  [unwired: 2 in, 2 out]
              }
              frame "Brightness  **", "Color Level  **", "Compression  **", "FPS  **", "Sharpness  **" {
                n165 = call <vilib>:"NT Read Number.vi"("Name"=w262) -> ("Numeric"=w261:dbl)  [unwired: 9 in, 1 out]
                n166 = local write "Test Slider"(w261) -> ()
                n167 = property on="Test Slider" class="Slide (strict)"("Visible"=TRUE, "Scale.Maximum"=100.0 ("Scale.Range:Maximum")) -> ()  [unwired: 2 in, 2 out]
                n168 = property on="Test Ring" class="Ring (strict)"("Visible"=FALSE) -> ()  [unwired: 2 in, 2 out]
              }
            }
          }
        }
        n169 = property on="Progress" class="Clust (strict)"("Visible"=FALSE) -> ()  [unwired: 2 in, 2 out]
      }
      event "Test Name": Mouse Enter {
        # "Populate the ring with the list of tests"
        n170 = event-data() -> ()  [unwired: 1 in, 1 out]
        n171 = call <vilib>:"NT Read String Array.vi"("Name"="TestMode/TestList") -> ("String Array"=w270:string[])  [unwired: 9 in, 1 out]
        n172 = Build Array (concatenate)("Select the test to run...", w270) -> (w269:string[])
        n173 = property on="Test Name" class="Ring (strict)"("Strings []"=w269) -> ()  [unwired: 2 in, 2 out]
      }
      event "Test Name": Value Change {
        w272 = FALSE ("Visible")
        # "Tell the robot the test name to run"
        n174 = event-data() -> ("NewVal"=w276:u16)  [unwired: 1 in]
        n175 = property on="Test Name" class="Ring (strict)"() -> ("Strings []"=w277:string[])  [unwired: 2 in, 2 out]
        n176 = local write "Progress"(T8 {"Test Progress"=0, "Test Progress Text"=""} ("Progress")) -> ()
        n177 = Index Array(array=w277, index=w276) -> (element=w275:string)
        n178 = call <vilib>:"NT Write String.vi"("String"=w275, "Name"="TestMode/TestName") -> ()  [unwired: 9 in, 1 out]
        n179 = property on="Progress" class="Clust (strict)"("Visible"=TRUE) -> ()  [unwired: 2 in, 2 out]
        n180 = property on="Motor" class="Clust (strict)"("Visible"=w272) -> ()  [unwired: 2 in, 2 out]
        n181 = property on="Test Slider" class="Slide (strict)"("Visible"=w272) -> ()  [unwired: 2 in, 2 out]
        n182 = property on="On/Off" class="Bool (strict)"("Visible"=w272) -> ()  [unwired: 2 in, 2 out]
        n183 = property on="Rev/Fwd" class="Clust (strict)"("Visible"=w272) -> ()  [unwired: 2 in, 2 out]
        n184 = property on="Test Ring" class="Ring (strict)"("Visible"=w272) -> ()  [unwired: 2 in, 2 out]
      }
      event "Listbox": Double Click {
        # "Shift clears all"
        # "Update symbols on the listbox"
        n185 = event-data() -> ("PlatMods.Shift"=w280:bool, "Row"=w282:i32)  [unwired: 1 in]
        n186 = case shown="True" w280 {
          tunnel: w282 -> [w286 _]
          tunnel: 1 -> [w285 _]
          frame False {
            n187 = property on="Listbox" class="LstBox (strict)"() -> ("Item Symbols"=w284:i32[])  [unwired: 2 in, 2 out]
            n188 = Replace Array Subset(array=w284, new element=w285, index=w286) -> (w283:i32[])
            n189 = property on="Listbox" class="LstBox (strict)"("Item Symbols"=w283) -> ()  [unwired: 2 in, 2 out]
          }
          frame True {
            w287 = 0 ("Top Row")
            n190 = property on="Listbox" class="LstBox (strict)"() -> ("Number of Rows"=w289:u32)  [unwired: 2 in, 2 out]
            n191 = Initialize Array(0, w289) -> (w288:i32[])
            n192 = property on="Listbox" class="LstBox (strict)"("Top Row"=w287, "Value"=w287, "Item Symbols"=w288) -> ()  [unwired: 2 in, 2 out]
          }
        }
      }
      event "Listbox": Key Down {
        # "Update symbols on the listbox\nLeft and right keys check and uncheck"
        n193 = event-data() -> ("VKey"=w293:T19)  [unwired: 1 in]
        n194 = case shown="\"Left\", \"Right\"" w293 {
          selector: w293 -> [w298 _]
          tunnel: eventvkey."Left" ("VKey") -> [w296 _]
          frame "Left", "Right" {
            n195 = Equal?(x=w296, y=w298) -> (x = y?=w297:bool)
            n196 = Select(t=0, s=w297, f=1) -> (s? t:f=w299:i32)
            n197 = property on="Listbox" class="LstBox (strict)"() -> ("Item Symbols"=w302:i32[])  [unwired: 2 in, 2 out]
            n198 = Replace Array Subset(array=w302, new element=w299, index="Listbox") -> (w301:i32[])
            n199 = property on="Listbox" class="LstBox (strict)"("Item Symbols"=w301) -> ()  [unwired: 2 in, 2 out]
          }
          frame Default {
          }
        }
      }
      event "DB Camera Config": Value Change {
        # "Show or hide the cluster of controls, store in ini file"
        n200 = event-data() -> ("NewVal"=w306:bool)  [unwired: 1 in]
        n201 = case shown="False" w306 {
          tunnel: w305 -> [w315 _]
          tunnel: [w308 w326] -> w304
          tunnel: w303 -> [w307 w326]
          frame False {
            w322 = "Camera"
            w325 = FALSE ("Visible")
            n202 = local read "Camera Settings"() -> (w314:T3)
            n203 = Index Array(array=w315) -> (element=w318:cluster{string[]})  [unwired: 1 in]
            n204 = Unbundle(w314) -> ("Frame Rate"=w313:i32, "Compression"=w312:i32, "Size"=w316:u16)
            n205 = Unbundle(w318) -> (w317:string[])
            n206 = Index Array(array=w317, index=w316) -> (element=w311:string)
            n207 = call-poly <vilib>:"Write Key.vi"("section"=w322, "value"=w311, "key"="Size", "refnum"=w307) -> ("refnum out"=w324:T17)  [unwired: 2 in, 5 out]
            n208 = call-poly <vilib>:"Write Key.vi"("section"=w322, "value"=w313, "key"="FrameRate", "refnum"=w324) -> ("refnum out"=w323:T17)  [unwired: 1 in, 6 out]
            n209 = property on="Camera Settings" class="Clust (strict)"("Visible"=w325) -> ()  [unwired: 2 in, 2 out]
            n210 = local write "DB Camera Config"(w325) -> ()
            n211 = call-poly <vilib>:"Write Key.vi"("section"=w322, "value"=w312, "key"="Compression", "refnum"=w323) -> ("refnum out"=w309:T17)  [unwired: 1 in, 6 out]
            n212 = call <vilib>:"Close Config Data.vi"("refnum"=w309) -> ("file path"=w310:path)  [unwired: 2 in, 8 out]
            n213 = call <vilib>:"Open Config Data.vi"("configuration file path"=w310) -> ("refnum"=w308:T17)  [unwired: 8 in, 2 out]
          }
          frame True {
            n214 = property on="Camera Settings" class="Clust (strict)"("Visible"=TRUE) -> ()  [unwired: 2 in, 2 out]
          }
        }
      }
      event "Camera Settings": Value Change {
        # "Update summary string when any elements of DB camera change"
        n215 = event-data() -> ("NewVal"=w339:T3)  [unwired: 1 in]
        n216 = Index Array(array=w335) -> (element=w334:cluster{string[]})  [unwired: 1 in]
        n217 = Unbundle(w339) -> ("Frame Rate"=w330:i32, "Compression"=w329:i32, "Size"=w332:u16)
        n218 = Unbundle(w334) -> (w333:string[])
        n219 = Index Array(array=w333, index=w332) -> (element=w331:string)
        n220 = Format Into String(format string="%s   %dfps   %d%%", w331, w330, w329) -> (resulting string=w336:string)  [unwired: 2 in, 1 out]
        n221 = Build Array(w336) -> (w337:string[])
        n222 = property on="DB Camera Config" class="Bool (strict)"("Strings [4]"=w337) -> ()  [unwired: 2 in, 2 out]
      }
      event "Motor.Enable": Value Change {
        # "When the test mode otor enable helper is set, update that\ntree row item's value"
        n223 = event-data() -> ("NewVal"=w345:bool)  [unwired: 1 in]
        n224 = Unbundle("Motor") -> ("Value"=w344:dbl)  [unwired: 1 out]
        n225 = Select(t=w344, s=w345, f=0.0) -> (s? t:f=w342:dbl)
        n226 = call <vilib>:"NT Write Number.vi"("Numeric"=w342, "Name"=w341) -> ()  [unwired: 9 in, 1 out]
      }
      event "Test Slider": Value Change {
        # "When the test mode slider helper is set, update that\ntree row item's value"
        n227 = event-data() -> ("NewVal"=w348:dbl)  [unwired: 1 in]
        n228 = call <vilib>:"NT Write Number.vi"("Numeric"=w348, "Name"=w349) -> ()  [unwired: 9 in, 1 out]
      }
      event "On/Off": Value Change {
        # "When the test mode on/off helper value is set, update that\ntree row item's value"
        n229 = event-data() -> ("NewVal"=w353:bool)  [unwired: 1 in]
        n230 = Boolean To (0,1)(Boolean=w353) -> (0, 1=w352:i16)
        n231 = call <vilib>:"NT Write Number.vi"("Numeric"=w352, "Name"=w351) -> ()  [unwired: 9 in, 1 out]
      }
      event "Rev/Fwd": Value Change {
        # "When the test mode helper value for relays is set, update that\ntree row item's value"
        n232 = event-data() -> ("NewVal.Forward"=w361:bool, "NewVal.Reverse"=w360:bool)  [unwired: 1 in]
        n233 = Boolean To (0,1)(Boolean=w361) -> (0, 1=w357:i16)
        n234 = Boolean To (0,1)(Boolean=w360) -> (0, 1=w359:i16)
        n235 = Negate(x=w359) -> (-x=w358:i16)
        n236 = Add(x=w357, y=w358) -> (x+y=w356:i16)
        n237 = call <vilib>:"NT Write Number.vi"("Numeric"=w356, "Name"=w355) -> ()  [unwired: 9 in, 1 out]
      }
      event "Test Ring": Value Change {
        # "When a test mode helper value is selected from the ring,\nset the tree item's variable to the string value"
        n238 = event-data() -> ("NewVal"=w365:u16)  [unwired: 1 in]
        n239 = property on="Test Ring" class="Ring (strict)"() -> ("Strings []"=w366:string[])  [unwired: 2 in, 2 out]
        n240 = Index Array(array=w366, index=w365) -> (element=w364:string)
        n241 = call <vilib>:"NT Write String.vi"("String"=w364, "Name"=w363) -> ()  [unwired: 9 in, 1 out]
      }
      event "Rec Mode": Value Change {
        # "Update globals for recording mode and path to read log from.\nClear when logging and let NetworkTables set path for vision to\nuse."
        n242 = event-data() -> ("NewVal"=w376:enum32{"Stop", "Record", "Playback"})  [unwired: 1 in]
        n243 = global write "WPI_DashboardLogging Global.vi" "Logging Filename"(path "") -> ()
        n244 = case shown="\"Playback\"" w376 {
          tunnel: w375 -> [_ w378 w386]
          tunnel: [_ _ w385] -> w372
          tunnel: [_ _ w384] -> _
          tunnel: w370 -> [_ _ w382]
          tunnel: cluster{i32, i32} {-250, 170} -> [_ _ w381]
          tunnel: [_ _ T20 {"Image Size"=TRUE, "Image Type"=TRUE, "Pixel Value"=TRUE, "ROI Information"=TRUE, "Zoom Factor"=FALSE} ("Image Information Shown:All Elements")] -> w368
          tunnel: [_ _ TRUE ("Zoom Factor")] -> w367
          frame Default {
          }
          frame "Stop", "Record" {
            # "Place Window too"
            n245 = invoke class="VI" method="FP.Close"(reference=w378) -> (reference out=w377:refnum<vi>)  [unwired: 2 in, 2 out]
            n246 = invoke class="VI" method="Abort VI"(reference=w377) -> ()  [unwired: 2 in, 3 out]
          }
          frame "Playback" {
            n247 = call "Open Playback Panel.vi"("Offset"=w381, "DB VI Ref"=w382, "Playback in"=w386) -> ("Playback out"=w383:refnum<vi>)  [unwired: 8 in]
            n248 = register-events(w383) -> (reference out=w385:refnum<event-registration>, error out=w384:errorcluster)  [unwired: 2 in]
          }
        }
        n249 = global write "WPI_DashboardLogging Global.vi" "Recording"(w376) -> ()
        n250 = property on="Camera Image" class="ImageControl"("Image Information Shown"=w368, "Image Information Visible"=w367) -> ()  [unwired: 2 in, 2 out]
        n251 = call <vilib>:"WPI_DashboardNT Log FieldName Cache.vi"("Operation"=enum16{"Lookup/Add", "Index", "Clear"}."Clear") -> ()  [unwired: 8 in, 3 out]
      }
      event Panel Close {
        w387 = enum32{"Stop", "Record", "Playback"}."Stop" ("Rec Mode")
        # "Playback window has been closed, abort"
        n252 = event-data() -> ()  [unwired: 1 in, 4 out]
        n253 = local write "Rec Mode"(w387) -> ()
        n254 = global write "WPI_DashboardLogging Global.vi" "Recording"(w387) -> ()
      }
      event Panel Close {
        # "Abort playback window and ourself"
        n255 = event-data() -> ()  [unwired: 1 in, 4 out]
        n256 = invoke class="VI" method="FP.Close"(reference=w392) -> (reference out=w391:refnum<vi>)  [unwired: 2 in, 2 out]
        n257 = invoke class="VI" method="Abort VI"(reference=w391) -> (error out=w390:errorcluster)  [unwired: 2 in, 2 out]
        n258 = invoke class="VI" method="Abort VI"(error in=w390) -> ()  [unwired: 2 in, 3 out]
      }
      event "Vision": Value Change {
        # "Enable/Disable Compression slider.\nHW USB is hard-coded into the camera"
        n259 = event-data() -> ("NewVal"=w398:u16)  [unwired: 1 in]
        n260 = Equal?(x=w398, y=u32 2 ("milliseconds to wait")) -> (x = y?=w396:bool)
        n261 = Select(t=T21."Disabled and Grayed Out" ("Disabled"), s=w396, f=T21."Enabled" ("Disabled")) -> (s? t:f=w393:T21)
        n262 = property on="Compression" class="Slide (strict)"("DisabledEnum"=w393) -> ()  [unwired: 2 in, 2 out]
      }
    }
  }
  n263 = while {
    tunnel: w35 -> [w401]
    i -> [w404]
    stop <- FALSE stop-if-true
    n264 = Wait (ms)(milliseconds to wait=u32 100) -> ()  [unwired: 1 out]
    n265 = case shown="\"Playback\"" "Rec Mode" {
      tunnel: w404 -> [_ _ w419]
      tunnel: [u32 2829099 ("Base Color") u32 11141120 ("Target Color") w408] -> w400
      frame "Stop", Default {
        # "Reset the color, extra updates don't cost much"
      }
      frame "Record" {
      }
      frame "Playback" {
        # "Playback"
        n266 = Quotient & Remainder(x=w419, y=u32 50 ("milliseconds to wait")) -> (x-y*floor(x/y)=w415:u32)  [unwired: 1 out]
        n267 = Divide(x=w415, y=u32 50 ("milliseconds to wait")) -> (x/y=w412:dbl)
        n268 = Multiply(x=6.283185307179586, y=w412) -> (x*y=w417:dbl)
        n269 = Sine(x=w417) -> (sin(x)=w416:dbl)
        n270 = Absolute Value(x=w416) -> (abs(x)=w409:dbl)
        n271 = call "Interpolate RGB Color.vi"("Proportion"=w409, "Target Color"=u32 30976, "Base Color"=u32 2829099) -> ("Result Color"=w408:u32)  [unwired: 8 in]
      }
    }
    n272 = property class="Pane"(reference=w401, "PaneColor"=w400) -> ()  [unwired: 1 in, 2 out]
  }
  n273 = TCP Create Listener(10:u16 1741 ("timeout ms (25000)")) -> (3:w3:refnum<k5>)  [unwired: 4 in, 2 out]
  n274 = while {
    tunnel: w3 -> [w421]
    stop <- FALSE stop-if-true
    n275 = TCP Wait On Listener(11:w421) -> (4:w420:refnum<k5>)  [unwired: 3 in, 4 out]
    n276 = local write "TCP"(w420) -> ()
  }
  n277 = property on="On/Off" class="Bool (strict)"("Visible"=w8) -> ()  [unwired: 2 in, 2 out]
  n278 = property on="Motor" class="Clust (strict)"("Visible"=w8) -> ()  [unwired: 2 in, 2 out]
  n279 = property on="Progress" class="Clust (strict)"("Visible"=w8) -> ()  [unwired: 2 in, 2 out]
  n280 = property on="Test Ring" class="Ring (strict)"("Visible"=w8) -> ()  [unwired: 2 in, 2 out]
  n281 = property on="Rev/Fwd" class="Clust (strict)"("Visible"=w8) -> ()  [unwired: 2 in, 2 out]
  n282 = property on="Camera Settings" class="Clust (strict)"("Visible"=w8) -> ()  [unwired: 2 in, 2 out]
  n283 = local write "DB Camera Config"(w8) -> ()
  n284 = global write "WPI_DashboardLogging Global.vi" "Recording"(w29) -> ()
  n285 = local write "Rec Mode"(w29) -> ()
